vi "Queue Reference (library variable).vi"() -> ()   [LabVIEW 2020, in "Error Manager.lvlib" / "MHL Queue.lvlib"]
uses:
  MHL Queue.lvlib
  Command (enum).ctl
  Message (cluster).ctl
panel:
  in  "Queue Reference":refnum<queue>
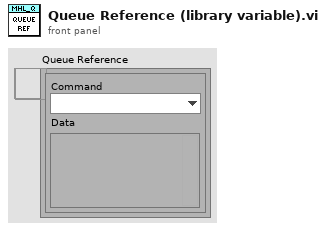
[diagram p1: front panel]
diagram:
